vi "TeleopCollisionDetection.vi"(10 "Match Info":T1={"Autonomous Elapsed Seconds"=0.0, "TeleOp Elapsed Seconds"=0.0, "Disabled Elapsed Seconds"=0.0, "Visited Autonomous"=FALSE, "Visited TeleOp"=FALSE, "Visited Disabled"=FALSE, "Autonomous Settings"={"Autonomous Style"=enum."Independent", "VI Refnum"=refnum}}, 11 "Call Context":T2) -> ()   [LabVIEW 2016]
doc: "This VI is called for each TeleOp packet received from the DS where the robot is not disabled. It is often used to read from the joysticks and update I/O or to update setpoints for timed control loops. It should complete and return within 20 milliseconds or it may miss DS packets."
uses:
  <vilib>/Rock Robotics/WPI/DriverStation/WPI_DriverStationDerivedRobotMode.ctl
  <vilib>/Rock Robotics/WPI/DriverStation/WPI_DriverStationMatch Info.ctl
  <vilib>/Rock Robotics/WPI/Utilities/WPI_GetSetVariantRefNum.vi
  <vilib>/Rock Robotics/Network Tables/SD Write Boolean.vi
  <vilib>/Rock Robotics/Network Tables/SD Write Numeric Array.vi
  <vilib>/Rock Robotics/Network Tables/SD Read Boolean.vi
  <vilib>/Rock Robotics/Network Tables/SD Read Number.vi
  <vilib>/Rock Robotics/WPI/RobotDrive/WPI_RobotDriveMecanumDrive_Cartesian.vi
panel:
  out "Sample Slider 0":dbl(slide) scale=0.0..5.0
  out "Sample Boolean 1":bool
  out "Sample Boolean 0":bool
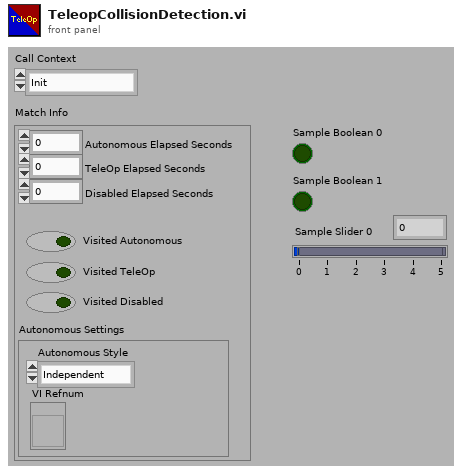
[diagram p1: front panel]
types:
  T1 = typedef "WPI_DriverStationMatch Info.ctl" = cluster{"Autonomous Elapsed Seconds":dbl, "TeleOp Elapsed Seconds":dbl, "Disabled Elapsed Seconds":dbl, "Visited Autonomous":bool, "Visited TeleOp":bool, "Visited Disabled":bool, "Autonomous Settings":cluster{"Autonomous Style":enum16{"Iterative", "Independent"}, "VI Refnum":refnum<vi>}}
  T2 = typedef "WPI_DriverStationDerivedRobotMode.ctl" = enum16{"Init", "Execute", "Stop"}
  T3 = cluster{"LinearAcceleration X":dbl, "LinearAcceleration Y":dbl, "LinearAcceleration Z":dbl}
  T4 = typedef "WPI_JoystickDevRef.ctl" = cluster{"Device":T5}
  T5 = typedef "WPI_JoystickDeviceEnum.ctl" = enum16{"USB 0", "USB 1", "USB 2", "USB 3", "USB 4", "USB 5"}
  T6 = typedef "WPI_RobotDriveDevRef.ctl" = cluster{"DevStatus":errorcluster, "Motors[]":T7[], "Square Inputs":bool, "Max Output":dbl}
  T7 = typedef "WPI_MotorControlDeviceRef.ctl" = cluster{"DeviceStatus":errorcluster, "Type":T8, "PWM":cluster{"PWM Channel":T9, "DeadBand":T10}, "CAN":cluster{"Device Number":u8, "SetOutput VI Ref":variant, "GetOutput VI Ref":variant, "Enable VI Ref":variant, "Disable VI Ref":variant, "Data":variant}, "Invert":bool}
  T8 = typedef "WPI_MotorControlType.ctl" = enum16{"PWM", "CAN"}
  T9 = typedef "FPGA_DIOPWMChannel.ctl" = enum8{"PWM 0", "PWM 1", "PWM 2", "PWM 3", "PWM 4", "PWM 5", "PWM 6", "PWM 7", "PWM 8", "PWM 9", "PWM MXP 0", "PWM MXP 1", "PWM MXP 2", "PWM MXP 3", "PWM MXP 4", "PWM MXP 5", "PWM MXP 6", "PWM MXP 7", "PWM MXP 8", "PWM MXP 9", "Invalid"}
  T10 = typedef "WPI_PWMDeadband.ctl" = cluster{"Name":string, "maxPositivePwm":i32, "minPositivePwm":i32, "centerPwm":i32, "maxNegativePwm":i32, "minNegativePwm":i32, "angularRange":u16}
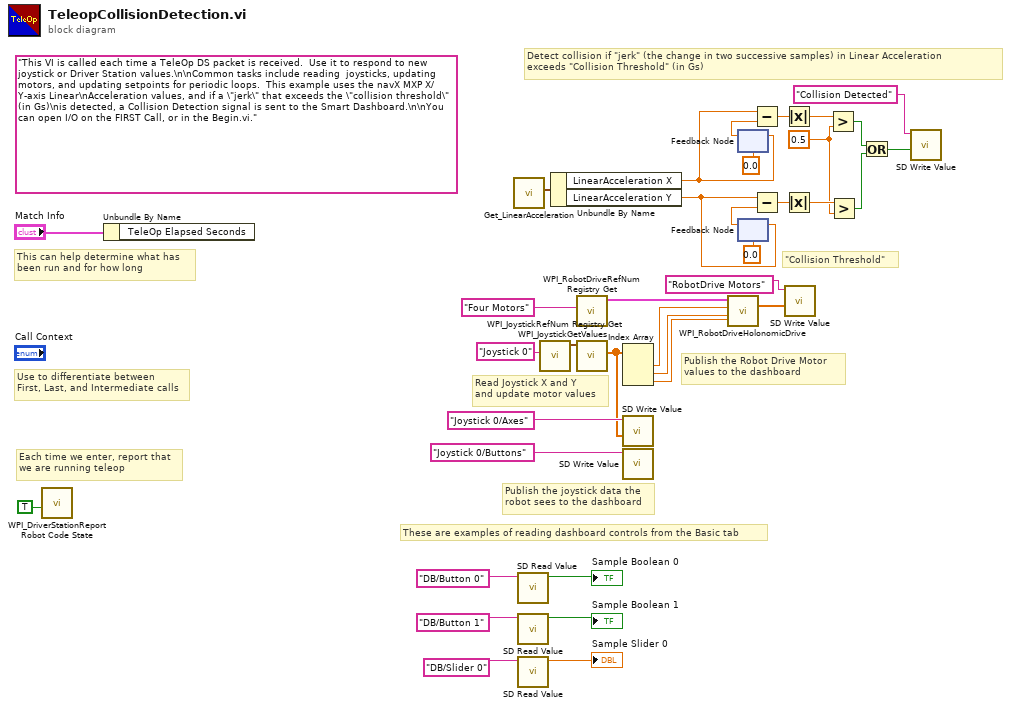
[diagram p0: block diagram]
diagram:
  w3 = 0.5
  (unwired) "This VI is called each time a TeleOp DS packet is received.  Use it to respond to new joystick or Driver Station values.\n\nCommon tasks include reading  joysticks, updating motors, and updating setpoints for periodic loops.  This example uses the navX MXP X/Y-axis Linear\nAcceleration values, and if a \"jerk\" that exceeds the \"collision threshold\" (in Gs)\nis detected, a Collision Detection signal is sent to the Smart Dashboard.\n\nYou can open I/O on the FIRST Call, or in the Begin.vi."
  # "\"Collision Threshold\""
  # "Detect collision if \"jerk\" (the change in two successive samples) in Linear Acceleration \nexceeds \"Collision Threshold\" (in Gs)"
  # "These are examples of reading dashboard controls from the Basic tab"
  # "Publish the Robot Drive Motor\nvalues to the dashboard"
  # "Publish the joystick data the\nrobot sees to the dashboard"
  # "Each time we enter, report that\nwe are running teleop"
  # "Use to differentiate between\nFirst, Last, and Intermediate calls"
  # "This can help determine what has\nbeen run and for how long"
  # "Read Joystick X and Y \nand update motor values"
  n1 = call <vilib>:"WPI_DriverStationReport Robot Code State.vi"("TeleOp"=TRUE ("Autonomous")) -> ()  [unwired: 10 in, 1 out]
  n2 = Unbundle By Name("Match Info") -> ()  [unwired: 1 out]
  n3 = call "Get_LinearAcceleration.vi"() -> ("Linear Acceleration"=w1:T3)  [unwired: 11 in]
  n4 = call-poly <vilib>:"SD Read Value.vi"("Name"="DB/Button 0" ("refnum name")) -> ("Boolean"=→"Sample Boolean 0":bool)  [unwired: 8 in, 2 out]
  n5 = call-poly <vilib>:"SD Read Value.vi"("Name"="DB/Button 1" ("refnum name")) -> ("Boolean"=→"Sample Boolean 1":bool)  [unwired: 8 in, 2 out]
  n6 = call-poly <vilib>:"SD Read Value.vi"("Name"="DB/Slider 0" ("refnum name")) -> ("Numeric"=→"Sample Slider 0":dbl)  [unwired: 8 in, 2 out]
  n7 = call <vilib>:"WPI_JoystickRefNum Registry Get.vi"("refnum name"="Joystick 0") -> ("JoystickDevRef"=w31:T4)  [unwired: 1 in, 9 out]
  n8 = Unbundle By Name(w1) -> ("LinearAcceleration X"=w12:dbl, "LinearAcceleration Y"=w2:dbl)
  n9 = call <vilib>:"WPI_RobotDriveRefNum Registry Get.vi"("refnum name"="Four Motors") -> ("RobotDriveDevRef"=w34:T6)  [unwired: 1 in, 9 out]
  n10 = call <vilib>:"WPI_JoystickGetValues.vi"("JoystickDevRef"=w31) -> ("Axes"=w17:dbl[])  [unwired: 6 in, 4 out]
  n11 = Index Array(array=w17) -> (element #1=w33:dbl, element #2=w19:dbl, element #3=w20:dbl)  [unwired: 3 in]
  n12 = call-poly <vilib>:"SD Write Value.vi"("Numeric Array"=w17, "Name"="Joystick 0/Axes") -> ()  [unwired: 8 in, 2 out]
  n13 = call-poly <vilib>:"SD Write Value.vi"("Name"="Joystick 0/Buttons") -> ()  [unwired: 9 in, 2 out]
  n14 = call-poly <vilib>:"WPI_RobotDriveHolonomicDrive.vi"("Rotation"=w20, "Y"=w19, "X"=w33, "RobotDriveDevRef"=w34) -> ("Motor Values"=w18:dbl[])  [unwired: 5 in, 2 out]
  n15 = feedback-in #1(w12) -> ()
  n16 = feedback #1(0.0) -> (w13:dbl)
  n17 = feedback #2(0.0) -> (w9:dbl)
  n18 = feedback-in #2(w2) -> ()
  n19 = Subtract(x=w12, y=w13) -> (x-y=w15:dbl)
  n20 = Subtract(x=w2, y=w9) -> (x-y=w7:dbl)
  n21 = Absolute Value(x=w15) -> (abs(x)=w14:dbl)
  n22 = Absolute Value(x=w7) -> (abs(x)=w8:dbl)
  n23 = call-poly <vilib>:"SD Write Value.vi"("Numeric Array"=w18, "Name"="RobotDrive Motors") -> ()  [unwired: 8 in, 2 out]
  n24 = Greater?(x=w14, y=w3) -> (0:w5:bool)
  n25 = Greater?(x=w8, y=w3) -> (0:w4:bool)
  n26 = Or(x=w5, y=w4) -> (x .or. y?=w11:bool)
  n27 = call-poly <vilib>:"SD Write Value.vi"("Boolean"=w11, "Name"="Collision Detected") -> ()  [unwired: 8 in, 2 out]
